vi "set_process_layer_parameters_cluster.vi"(6 "Process layer parameters":T1, 8 "error in (no error)":errorcluster, 9 "Layer number":u8, 10 "Process number":u8, 11 "VISA resource name":refnum<visa-resource-name>) -> (0 "error out":errorcluster, 3 "VISA resource name out":refnum<visa-resource-name>)   [LabVIEW 2018]
doc: "Set the density of a material."
uses:
  Low Level/process_layer_parameters.ctl
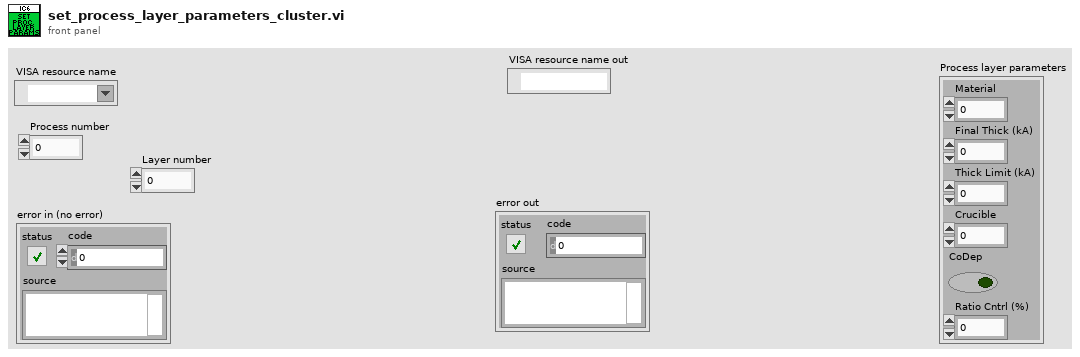
[diagram p1: front panel]
types:
  T1 = typedef "process_layer_parameters.ctl" = cluster{"Material":u8, "Final Thick (kA)":sgl, "Thick Limit (kA)":sgl, "Crucible":u8, "CoDep":bool, "Ratio Cntrl (%)":sgl}
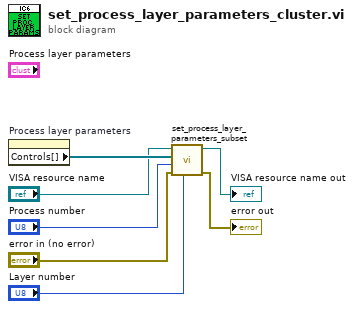
[diagram p0: block diagram]
diagram:
  n1 = property on="Process layer parameters" class="Clust (strict)"() -> ("Controls[]"=w3:refnum<vi>[])  [unwired: 2 in, 2 out]
  n2 = call "set_process_layer_parameters_subset.vi"("Layer number"="Layer number", "error in (no error)"="error in (no error)", "Process number"="Process number", "Controls[]"=w3, "VISA resource name"="VISA resource name") -> ("error out"=→"error out":errorcluster, "VISA Refnum out"=→"VISA resource name out":refnum<visa-resource-name>)  [unwired: 5 in]
